vi "test2.vi"() -> ()   [LabVIEW 2019]
uses:
  <vilib>/rvi/Emulation/niFpgaGetClockAttributes.vi
  <vilib>/rvi/Emulation/niFpgaSctlEmulationGetInTimedLoop.vi
  <vilib>/rvi/Emulation/niFpgaEmulationReportErrorSimple.vi
  <vilib>/rvi/eio/common/nirviEmuTemplateMethod_errors.vi
  <vilib>/rvi/Emulation/niFpgaCriticalErrorInLSC.vi
  <vilib>/eio/EIONode/EIONode.xnode
panel:
  in  "stop":bool
  out "AccelerationZ":i16
  out "AccelerationY":i16
  out "AccelerationX":i16
  in  "Seuil z":i16
  in  "Seuil y":i16
  in  "Seuil x":i16
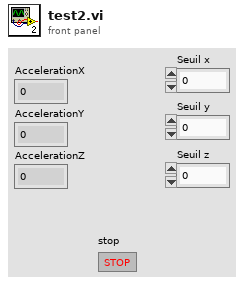
[diagram p1: front panel]
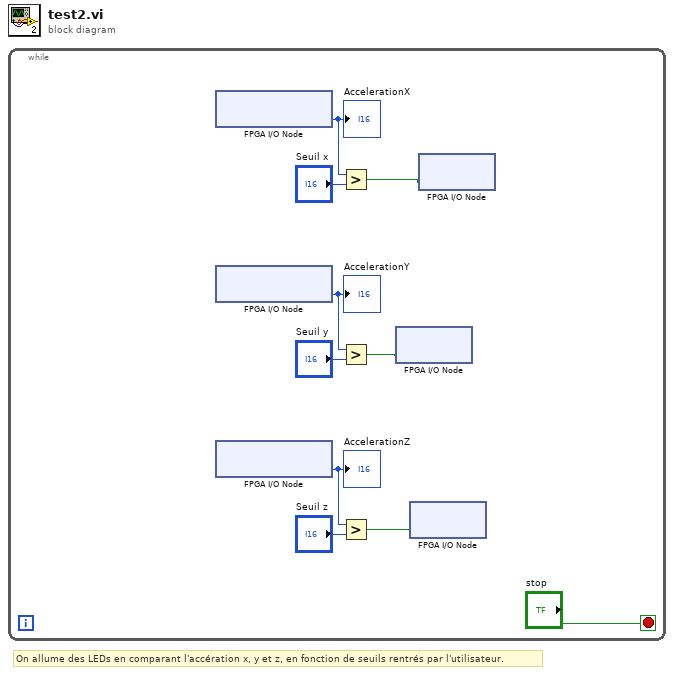
[diagram p0: block diagram]
diagram:
  # "On allume des LEDs en comparant l'accération x, y et z, en fonction de seuils rentrés par l'utilisateur."
  n1 = while {
    stop <- "stop" stop-if-true
    n2 = xnode "FPGA I/O Node"() -> ("AccelerationX"=w9:i16)  [unwired: 1 in, 1 out]
    "AccelerationX" <- w9
    n3 = xnode "FPGA I/O Node"() -> ("AccelerationY"=w8:i16)  [unwired: 1 in, 1 out]
    "AccelerationY" <- w8
    n4 = xnode "FPGA I/O Node"() -> ("AccelerationZ"=w6:i16)  [unwired: 1 in, 1 out]
    "AccelerationZ" <- w6
    n5 = Greater?(x=w9, y="Seuil x") -> (0:w4:bool)
    n6 = Greater?(x=w8, y="Seuil y") -> (0:w3:bool)
    n7 = Greater?(x=w6, y="Seuil z") -> (0:w2:bool)
    n8 = xnode "FPGA I/O Node"("LED1"=w3) -> ()  [unwired: 1 in, 1 out]
    n9 = xnode "FPGA I/O Node"("LED2"=w2) -> ()  [unwired: 1 in, 1 out]
    n10 = xnode "FPGA I/O Node"("LED0"=w4) -> ()  [unwired: 1 in, 1 out]
  }
